vi "get_raster_input_meta_data.vi"(11 "Path":path) -> (2 "cluster":T1)   [LabVIEW 2017]
uses:
  controls/raster_input_meta_data.ctl
  <vilib>/Platform/storage/lvStorage.llb/_openFunction.ctl
  <vilib>/Platform/storage/lvStorage.llb/_openStorageWithRootAutoDetect.vi
  <vilib>/Platform/storage/lvStorage.llb/xStorage/xStorageSupp/ErrorOut.vi
  <vilib>/Platform/storage/lvStorage.llb/_queryPropPoly.vi
  <vilib>/Platform/storage/lvStorage.llb/_queryPropString.vi
  <vilib>/Platform/storage/lvStorage.llb/_queryGenericObjects.vi
  <vilib>/Platform/storage/lvStorage.llb/_loadAllDdt.vi
  <vilib>/Platform/storage/lvStorage.llb/xStorage/Open Data Storage/Open Data Storage.xnode
  <vilib>/Platform/storage/lvStorage.llb/xStorage/Read Data/Read Data.xnode
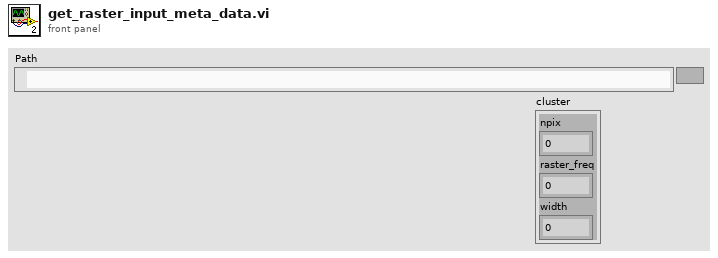
[diagram p1: front panel]
types:
  T1 = typedef "raster_input_meta_data.ctl" = cluster{"npix":dbl, "raster_freq":dbl, "width":dbl}
  T2 = typedef "usiPluginInformation.ctl" = cluster{"name":string, "version":string, "type":string, "read-only?":bool, "extensions":string[]}
  T3 = enum16{"UPDATE", "READ", "QUERY", "CREATE CHILD", "CREATE", "CONNECT", "DISCONNECT"}
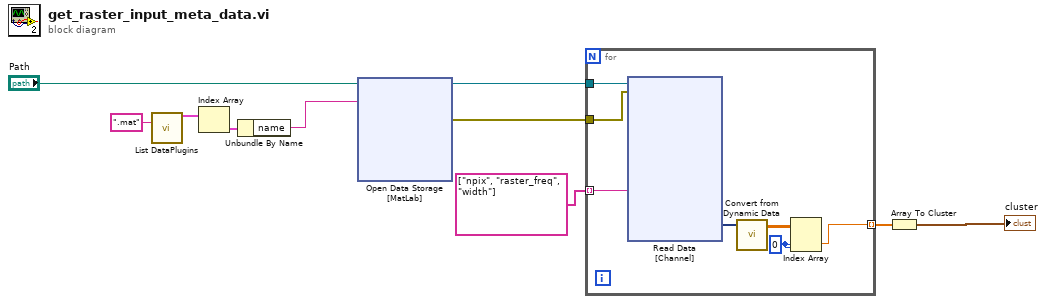
[diagram p0: block diagram]
diagram:
  n1 = call <vilib>:"List DataPlugins.vi"("file extension"=".mat") -> ("DataPlugin information"=w8:T2[])  [unwired: 13 in, 1 out]
  n2 = Index Array(array=w8) -> (element=w7:T2)  [unwired: 1 in]
  n3 = Unbundle By Name(w7) -> ("name"=w6:string)
  n4 = xnode "Open Data Storage\n[MatLab]"("file path"="Path", "DataPlugin name"=w6) -> ("storage refnum (file)"=w4:refnum<k20>, "error out"=w5:errorcluster)  [unwired: 3 in, 1 out]
  n5 = for {
    tunnel: w5 -> [w17]
    tunnel: w4 -> [w16]
    tunnel: string[] ["npix", "raster_freq", "width"] -> [w14] mode=indexing
    tunnel: [w12] -> w1 mode=indexing
    w11 = 0 ("index (row)")
    n6 = xnode "Read Data\n[Channel]"("Name"=w14, "storage refnum (file)"=w16, "error in"=w17) -> ("Signal"=w15:dynamicdata)  [unwired: 3 in, 3 out]
    n7 = call "Convert from Dynamic Data"("Dynamic Data Type"=w15) -> ("Array"=w13:dbl[][])  [unwired: 3 in]
    n8 = Index Array(array=w13, index (row)=w11, index (col)=w11) -> (element=w12:dbl)
  }
  n9 = Array To Cluster(array=w1) -> (cluster=→"cluster":cluster{"[0]":dbl, "[1]":dbl, "[2]":dbl})
